vi "Semaphore Unlock.vi"(11 "semaphore":refnum<queue>) -> ()   [LabVIEW 2017, in "CSM Shared.lvlib"]
uses:
  CSM Shared.lvlib
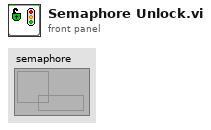
[diagram p1: front panel]
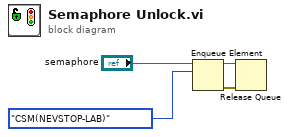
[diagram p0: block diagram]
diagram:
  n1 = Enqueue Element(queue="semaphore", element=enum16{"CSM(NEVSTOP-LAB)"}."CSM(NEVSTOP-LAB)") -> (queue out=w2:refnum<queue>, error out=w3:errorcluster)  [unwired: 2 in, 1 out]
  n2 = Release Queue(queue=w2, error in (no error)=w3) -> ()  [unwired: 1 in, 3 out]
